vi "ArmGetPresets.vi"(10 "Game Piece":T2, 11 "Position":T1=enum."Middle") -> (1 "z":dbl, 3 "x":dbl)   [LabVIEW 2020]
uses:
  ArmGamePiecePreset.ctl
  ArmPositionPreset.ctl
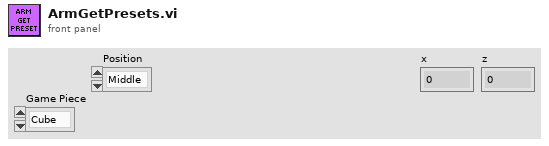
[diagram p1: front panel]
types:
  T1 = typedef "ArmPositionPreset.ctl" = enum16{"Upper", "Lower", "Middle", "Shelf", "Floor"}
  T2 = typedef "ArmGamePiecePreset.ctl" = enum16{"Cube", "Cone"}
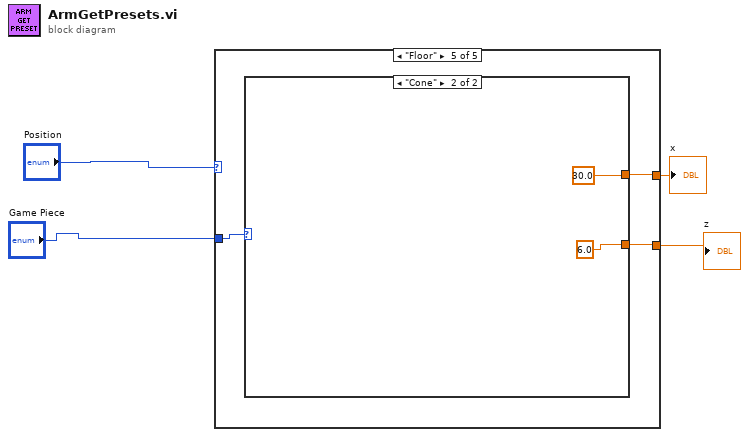
[diagram p0: block diagram]
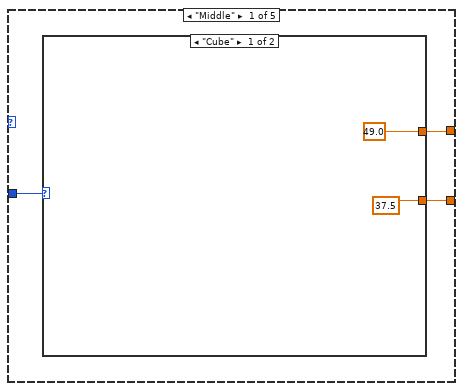
[diagram p2: hidden frame]
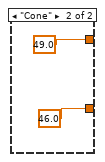
[diagram p3: hidden frame]
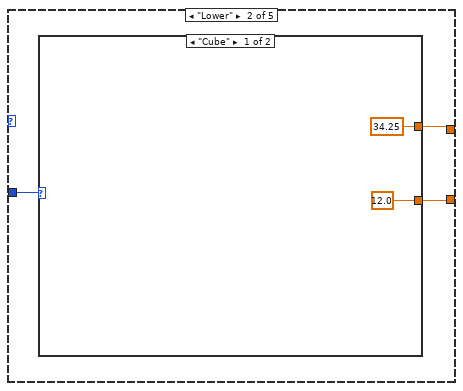
[diagram p4: hidden frame]
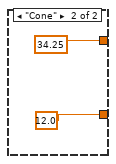
[diagram p5: hidden frame]
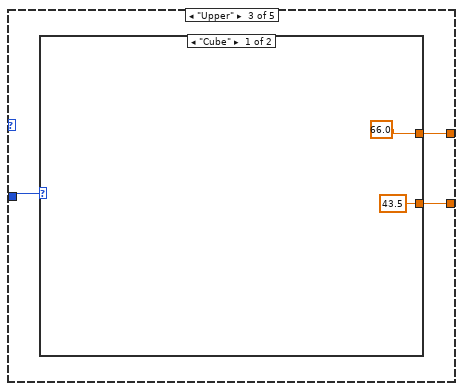
[diagram p6: hidden frame]
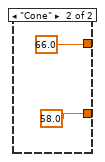
[diagram p7: hidden frame]
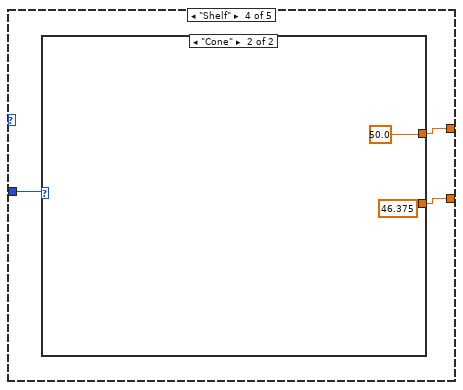
[diagram p8: hidden frame]
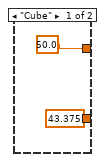
[diagram p9: hidden frame]
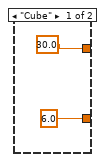
[diagram p10: hidden frame]
diagram:
  n1 = case shown="\"Floor\"" "Position" {
    tunnel: [w6 w14 w21 w27 w35] -> w4
    tunnel: [w5 w13 w20 w26 w34] -> w3
    tunnel: "Game Piece" -> [w7 w12 w19 w28 w33]
    frame "Middle" {
      n2 = case shown="\"Cube\"" w7 {
        tunnel: [49.0 49.0] -> w6
        tunnel: [37.5 46.0] -> w5
        frame "Cube" {
        }
        frame "Cone" {
        }
      }
    }
    frame "Lower" {
      n3 = case shown="\"Cube\"" w12 {
        tunnel: [34.25 34.25] -> w14
        tunnel: [12.0 12.0] -> w13
        frame "Cube" {
        }
        frame "Cone" {
        }
      }
    }
    frame "Upper" {
      n4 = case shown="\"Cube\"" w19 {
        tunnel: [66.0 66.0] -> w21
        tunnel: [43.5 58.0] -> w20
        frame "Cube" {
        }
        frame "Cone" {
        }
      }
    }
    frame "Shelf" {
      n5 = case shown="\"Cone\"" w28 {
        tunnel: [50.0 50.0] -> w27
        tunnel: [43.375 46.375] -> w26
        frame "Cube" {
        }
        frame "Cone" {
        }
      }
    }
    frame "Floor" {
      n6 = case shown="\"Cone\"" w33 {
        tunnel: [30.0 30.0] -> w35
        tunnel: [6.0 6.0] -> w34
        frame "Cube" {
        }
        frame "Cone" {
        }
      }
    }
  }
  "x" <- w4
  "z" <- w3
